vi "GUI.vi"() -> ()   [LabVIEW 2014]
panel:
  in  "?":T1(tab)
  out "Upozorenja":cluster{"H3":bool, "H5":bool, "H7":bool}
  out "Nadziranje":T2
  in  "Upravljanje":cluster{"Total_stop":bool, "Start":bool}
  out "Indikatori rada motora":T3
  out "Senzori":T4
  # "Skladište malih paketa je popunjeno!"
  # "Skladište srednjih paketa je popunjeno!"
  # "Skladište velikih paketa je popunjeno!"
  # "Prva traka"
  # "Traka za prvi sprat"
  # "Traka za drugi sprat"
  # "Traka za treci sprat"
  # "Lift traka"
  # "Lift - DOLE"
  # "Lift - GORE"
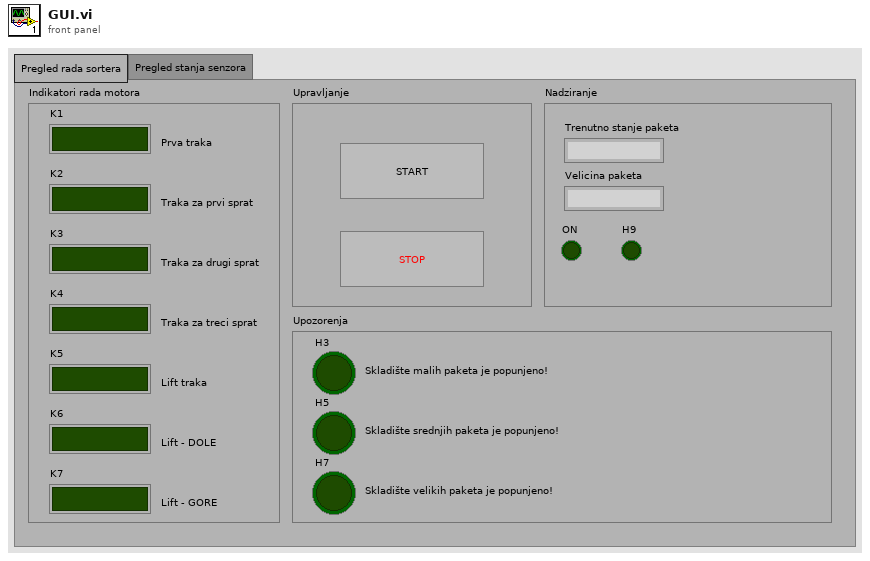
[diagram p1: front panel]
types:
  T1 = enum32{"Pregled rada sortera", "Pregled stanja senzora"}
  T2 = cluster{"Trenutno stanje paketa":string, "Velicina paketa":string, "ON":bool, "H9":bool}
  T3 = cluster{"K1":bool, "K2":bool, "K3":bool, "K4":bool, "K5":bool, "K6":bool, "K7":bool}
  T4 = cluster{"B1":bool, "B2":bool, "B3":bool, "B4":bool, "B5":bool, "B6":bool, "B7":bool, "B8":bool, "B9":bool, "B10":bool, "B11":bool}
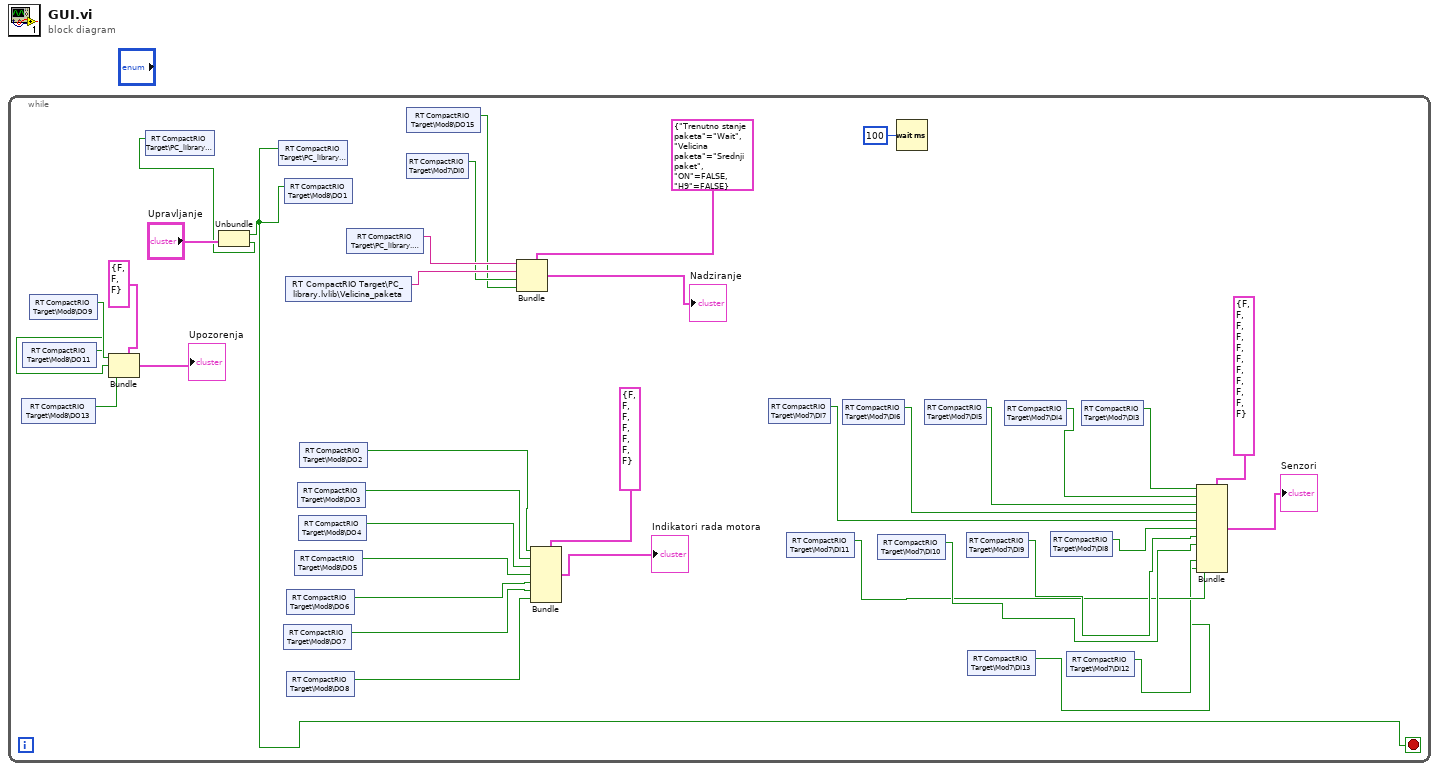
[diagram p0: block diagram]
diagram:
  n1 = while {
    stop <- w6 stop-if-true
    n2 = shared-variable "RT CompactRIO Target\\Mod8\\DO13"() -> (w8:bool)  [unwired: 1 in, 1 out]
    n3 = shared-variable "RT CompactRIO Target\\Mod8\\DO11"() -> (w9:bool)  [unwired: 1 in, 1 out]
    n4 = shared-variable "RT CompactRIO Target\\Mod8\\DO9"() -> (w10:bool)  [unwired: 1 in, 1 out]
    n5 = Bundle(cluster=cluster{"H3":bool, "H5":bool, "H7":bool} {"H3"=FALSE, "H5"=FALSE, "H7"=FALSE} ("Upozorenja"), "H3"=w10, "H5"=w9, "H7"=w8) -> (→"Upozorenja":cluster{"H3":bool, "H5":bool, "H7":bool})
    n6 = Unbundle("Upravljanje") -> ("Total_stop"=w6:bool, "Start"=w30:bool)
    n7 = shared-variable "RT CompactRIO Target\\PC_library.lvlib\\Start"(w30) -> ()  [unwired: 1 in, 1 out]
    n8 = shared-variable "RT CompactRIO Target\\PC_library.lvlib\\Stop"(w6) -> ()  [unwired: 1 in, 1 out]
    n9 = shared-variable "RT CompactRIO Target\\Mod8\\DO7"() -> (w13:bool)  [unwired: 1 in, 1 out]
    n10 = shared-variable "RT CompactRIO Target\\Mod8\\DO1"(w6) -> ()  [unwired: 1 in, 1 out]
    n11 = shared-variable "RT CompactRIO Target\\PC_library.lvlib\\Velicina_paketa"() -> (w31:string)  [unwired: 1 in, 1 out]
    n12 = shared-variable "RT CompactRIO Target\\Mod8\\DO6"() -> (w14:bool)  [unwired: 1 in, 1 out]
    n13 = shared-variable "RT CompactRIO Target\\Mod8\\DO8"() -> (w12:bool)  [unwired: 1 in, 1 out]
    n14 = shared-variable "RT CompactRIO Target\\Mod8\\DO5"() -> (w15:bool)  [unwired: 1 in, 1 out]
    n15 = shared-variable "RT CompactRIO Target\\Mod8\\DO3"() -> (w17:bool)  [unwired: 1 in, 1 out]
    n16 = shared-variable "RT CompactRIO Target\\Mod8\\DO4"() -> (w16:bool)  [unwired: 1 in, 1 out]
    n17 = shared-variable "RT CompactRIO Target\\Mod8\\DO2"() -> (w18:bool)  [unwired: 1 in, 1 out]
    n18 = shared-variable "RT CompactRIO Target\\PC_library.lvlib\\Stanje"() -> (w32:string)  [unwired: 1 in, 1 out]
    n19 = shared-variable "RT CompactRIO Target\\Mod8\\DO15"() -> (w3:bool)  [unwired: 1 in, 1 out]
    n20 = shared-variable "RT CompactRIO Target\\Mod7\\DI0"() -> (w4:bool)  [unwired: 1 in, 1 out]
    n21 = Bundle(cluster=T2 {"Trenutno stanje paketa"="Wait", "Velicina paketa"="Srednji paket", "ON"=FALSE, "H9"=FALSE} ("Nadziranje"), "Trenutno stanje paketa"=w32, "Velicina paketa"=w31, "ON"=w4, "H9"=w3) -> (→"Nadziranje":T2)
    n22 = Bundle(cluster=T3 {"K1"=FALSE, "K2"=FALSE, "K3"=FALSE, "K4"=FALSE, "K5"=FALSE, "K6"=FALSE, "K7"=FALSE} ("Indikatori rada motora"), "K1"=w18, "K2"=w17, "K3"=w16, "K4"=w15, "K5"=w14, "K6"=w13, "K7"=w12) -> (→"Indikatori rada motora":T3)
    n23 = shared-variable "RT CompactRIO Target\\Mod7\\DI7"() -> (w25:bool)  [unwired: 1 in, 1 out]
    n24 = shared-variable "RT CompactRIO Target\\Mod7\\DI11"() -> (w21:bool)  [unwired: 1 in, 1 out]
    n25 = shared-variable "RT CompactRIO Target\\Mod7\\DI6"() -> (w29:bool)  [unwired: 1 in, 1 out]
    n26 = shared-variable "RT CompactRIO Target\\Mod7\\DI10"() -> (w22:bool)  [unwired: 1 in, 1 out]
    n27 = Wait (ms)(milliseconds to wait=u32 100) -> ()  [unwired: 1 out]
    n28 = shared-variable "RT CompactRIO Target\\Mod7\\DI5"() -> (w26:bool)  [unwired: 1 in, 1 out]
    n29 = shared-variable "RT CompactRIO Target\\Mod7\\DI9"() -> (w23:bool)  [unwired: 1 in, 1 out]
    n30 = shared-variable "RT CompactRIO Target\\Mod7\\DI13"() -> (w19:bool)  [unwired: 1 in, 1 out]
    n31 = shared-variable "RT CompactRIO Target\\Mod7\\DI4"() -> (w27:bool)  [unwired: 1 in, 1 out]
    n32 = shared-variable "RT CompactRIO Target\\Mod7\\DI8"() -> (w24:bool)  [unwired: 1 in, 1 out]
    n33 = shared-variable "RT CompactRIO Target\\Mod7\\DI12"() -> (w20:bool)  [unwired: 1 in, 1 out]
    n34 = shared-variable "RT CompactRIO Target\\Mod7\\DI3"() -> (w28:bool)  [unwired: 1 in, 1 out]
    n35 = Bundle(cluster=T4 {"B1"=FALSE, "B2"=FALSE, "B3"=FALSE, "B4"=FALSE, "B5"=FALSE, "B6"=FALSE, "B7"=FALSE, "B8"=FALSE, "B9"=FALSE, "B10"=FALSE, "B11"=FALSE} ("Senzori"), "B1"=w28, "B2"=w27, "B3"=w26, "B4"=w29, "B5"=w25, "B6"=w24, "B7"=w23, "B8"=w22, "B9"=w21, "B10"=w20, "B11"=w19) -> (→"Senzori":T4)
  }
